vi "RH_DCPower_Fetch.vi"(7 "Wait":bool, 8 "error in (no error)":errorcluster, 9 "NumSamples":i32=1 caption="count (1)", 10 "channel name":string, 11 "DCPower Session In":refnum<k15>) -> (0 "error out":errorcluster, 1 "Current":dbl[](array[numeric]), 2 "Voltage":dbl[](array[numeric]), 3 "DCPower Session Out":refnum<k15>)   [LabVIEW 2023, in "ResourceHandling.lvlib"]
doc: "Fetches NumSamples of Voltage and Current"
uses:
  ResourceHandling.lvlib
  <instrlib>/niDCPower/nidcpower.llb/niDCPower Wait For Event - Event.ctl
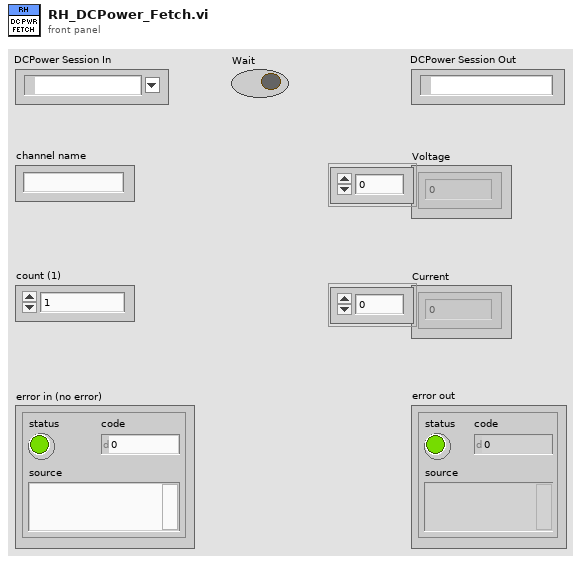
[diagram p1: front panel]
types:
  T1 = typedef "niDCPower Wait For Event - Event.ctl" = i32
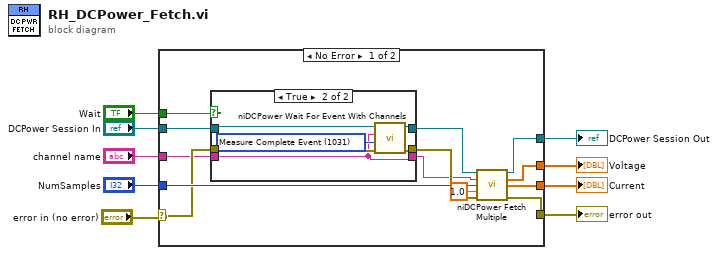
[diagram p0: block diagram]
diagram:
  n1 = case shown="No Error" "error in (no error)" {
    selector: "error in (no error)" -> [w15 w32]
    tunnel: [w22 w32] -> w9
    tunnel: [w21 w33] -> w2
    tunnel: "DCPower Session In" -> [w17 w33]
    tunnel: "NumSamples" -> [w20 _]
    tunnel: [w19 _] -> w6
    tunnel: [w18 _] -> w5
    tunnel: "channel name" -> [w11 _]
    tunnel: "Wait" -> [w14 _]
    frame No Error {
      n2 = case shown="True" w14 {
        tunnel: w17 -> [w25 w31]
        tunnel: [w25 w30] -> w16
        tunnel: [w24 w29] -> w12
        tunnel: w15 -> [w24 w28]
        tunnel: w11 -> [w23 w26]
        tunnel: [w23 w26] -> w10
        frame False {
        }
        frame True {
          w27 = T1 1031 items=["Source Complete Event"=1030, "Measure Complete Event"=1031, "Sequence Iteration Complete Event"=1032, "Sequence Engine Done Event"=1033, "Pulse Complete Event"=1051, "Ready For Pulse Trigger Event"=1052] ("event")
          n3 = call <instrlib>:"niDCPower Wait For Event With Channels.vi"("error in (no error)"=w28, "event"=w27, "channel name"=w26, "instrument handle"=w31) -> ("error out"=w29:errorcluster, "instrument handle out"=w30:refnum<k15>)  [unwired: 6 in]
        }
      }
      n4 = call <instrlib>:"niDCPower Fetch Multiple.vi"("instrument handle"=w16, "channel name"=w10, "count (1)"=w20, "timeout (1.0)"=1.0 ("timeout (sec)"), "error in (no error)"=w12) -> ("instrument handle out"=w21:refnum<k15>, "voltage measurements"=w19:dbl[], "current measurements"=w18:dbl[], "error out"=w22:errorcluster)  [unwired: 5 in, 2 out]
    }
    frame Error {
    }
  }
  "error out" <- w9
  "Voltage" <- w6
  "Current" <- w5
  "DCPower Session Out" <- w2
